vi "Notify.vi"(8 "Error In":errorcluster, 10 "Message":string, 11 "reference in":refnum<class "Tester.lvclass">) -> (0 "Error Out":errorcluster, 3 "reference in":refnum<class "Tester.lvclass">)   [LabVIEW 2020, in "Tester.lvclass"]
uses:
  Tester.lvclass
  Console_class/Console.lvclass
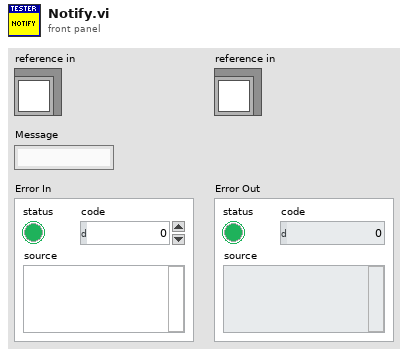
[diagram p1: front panel]
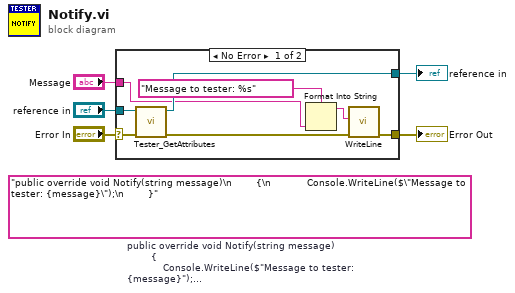
[diagram p0: block diagram]
diagram:
  (unwired) "public override void Notify(string message)\n        {\n            Console.WriteLine($\"Message to tester: {message}\");\n        }"  # public override void Notify(string message)         {             Console.WriteLine($"Message to tester: {message}");         }
  n1 = case shown="No Error" "Error In" {
    selector: "Error In" -> [w12 w15]
    tunnel: [w7 w15] -> w4
    tunnel: [w11 w14] -> w2
    tunnel: "reference in" -> [w13 w14]
    tunnel: "Message" -> [w6 _]
    frame No Error {
      n2 = call "Tester_GetAttributes.vi"("error in (no error)"=w12, "reference in"=w13) -> ("error out"=w8:errorcluster, "reference out"=w11:refnum<class "Tester.lvclass">)  [unwired: 6 in, 2 out]
      n3 = Format Into String(format string="Message to tester: %s", w6) -> (resulting string=w9:string)  [unwired: 2 in, 1 out]
      n4 = call "WriteLine.vi"("Error In"=w8, "ConsoleText"=w9) -> ("Error Out"=w7:errorcluster)  [unwired: 9 in]
    }
    frame Error {
    }
  }
  "Error Out" <- w4
  "reference in" <- w2
